vi "write IP configuration.vi"(7 "gateway":string, 8 "error in (no error)":errorcluster, 9 "subnet_mask":string, 10 "IP":string, 11 "identifier":string) -> (0 "error out":errorcluster, 1 "subnet_mask out":string, 2 "IP out":string, 3 "function return":u32, 5 "gateway out":string)   [LabVIEW 2015, in "XGL_DPP.lvlib"]
doc: "EXTERN DECLSPEC uint32_t CALL_CONV write_IP_configuration(const char * identifier, char * IP, char * subnet_mask, char * gateway);"
uses:
  XGL_DPP.lvlib
  XGL_DPP.dll
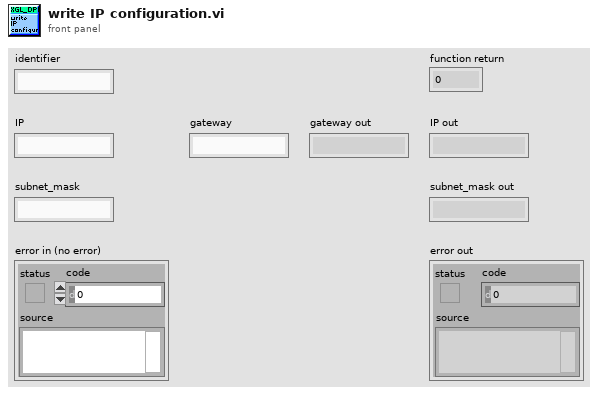
[diagram p1: front panel]
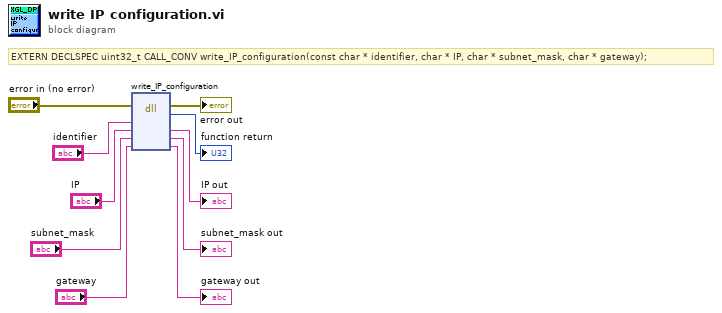
[diagram p0: block diagram]
diagram:
  # "EXTERN DECLSPEC uint32_t CALL_CONV write_IP_configuration(const char * identifier, char * IP, char * subnet_mask, char * gateway);"
  n1 = dll-call lib="D:/Users/XRF/Desktop/Scanning Software_Demokritos_2015_v7/libs/Vis_2/XGL_DPP.*" fn="write_IP_configuration"(error in="error in (no error)", "identifier"="identifier", "IP"="IP", "subnet_mask"="subnet_mask", "gateway"="gateway") -> (error out=→"error out":errorcluster, →"function return":u32, "IP"=→"IP out":string, "subnet_mask"=→"subnet_mask out":string, "gateway"=→"gateway out":string)  [unwired: 3 in, 1 out]
